vi "Show Main VI.vi"   [LabVIEW 2016]
types:
  T1 = enum32{"Invalid", "Standard", "Closed", "Hidden", "Minimized", "Maximized"}
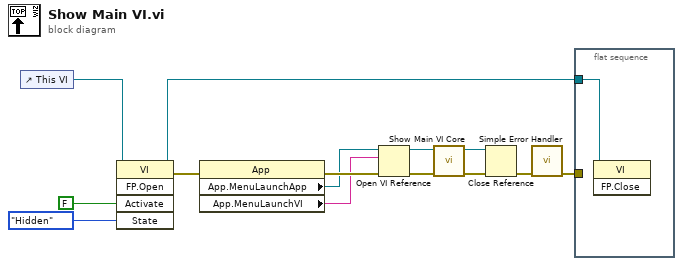
[diagram p0: block diagram]
diagram:
  n1 = control-ref of="This VI"() -> (w14:refnum<vi>)
  n2 = invoke class="VI" method="FP.Open"(reference=w14, "Activate"=FALSE ("Activate?"), "State"=T1."Hidden") -> (reference out=w11:refnum<vi>, error out=w12:errorcluster)  [unwired: 2 in, 3 out]
  n3 = property class="App"(error in=w12) -> (error out=w8:errorcluster, "App.MenuLaunchApp"=w7:refnum<vi>, "App.MenuLaunchVI"=w6:string)  [unwired: 1 in, 1 out]
  n4 = Open VI Reference(application reference (local)=w7, vi path=w6, error in (no error)=w8) -> (vi reference=w3:refnum<vi>, error out=w4:errorcluster)  [unwired: 3 in]
  n5 = call "Show Main VI Core.vi"("error in (no error)"=w4, "Calling VI Ref in"=w3) -> ("error out"=w2:errorcluster, "Calling VI Ref out"=w1:refnum<vi>)  [unwired: 8 in]
  n6 = Close Reference(reference=w1, error in (no error)=w2) -> (error out=w5:errorcluster)
  n7 = call <vilib>:"Simple Error Handler.vi"("error in (no error)"=w5) -> ("error out"=w9:errorcluster)  [unwired: 4 in, 4 out]
  n8 = flat-sequence {
    tunnel: w11 -> [w15]
    tunnel: w9 -> [_]
    frame #0 {
      n9 = invoke class="VI" method="FP.Close"(reference=w15) -> ()  [unwired: 2 in, 3 out]
    }
  }
